vi "Write Datalog file pathname.vi"(1 "Datalog file pathname.":path) -> (0 "PASS/FAIL.":bool)   [LabVIEW 2010]
panel:
  # "Inputs:"
  # "Outputs."
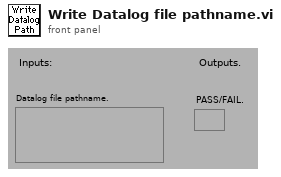
[diagram p1: front panel]
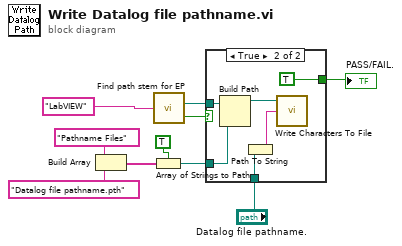
[diagram p0: block diagram]
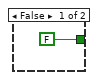
[diagram p2: hidden frame]
diagram:
  n1 = Build Array("Pathname Files", "Datalog file pathname.pth") -> (w7:string[])
  n2 = Array of Strings to Path(0:w7, 1:TRUE) -> (2:w10:path)
  n3 = call "Find path stem for EP.vi"("Node of path stem."="LabVIEW") -> ("Path stem."=w8:path, "PASS/FAIL"=w9:bool)
  n4 = case shown="True" w9 {
    tunnel: w8 -> [_ w17]
    tunnel: w10 -> [_ w16]
    tunnel: [FALSE TRUE] -> w2
    tunnel: "Datalog file pathname." -> [_ w12]
    frame False {
    }
    frame True {
      n5 = Build Path(base path=w17, name or relative path=w16) -> (appended path=w14:path)
      n6 = Path To String(path=w12) -> (string=w13:string)
      n7 = call <vilib>:"Write Characters To File.vi"("character string"=w13, "file path (dialog if empty)"=w14) -> ()  [unwired: 1 in, 3 out]
    }
  }
  "PASS/FAIL." <- w2
